vi "IO Docs.vi"(6 "OffsetGain":dbl[](array[numeric]), 7 "User Creds":T1, 8 "Error In":errorcluster, 9 "Digital IO":bool[](array[boolean]), 11 "Analog IO":dbl[](array[numeric])) -> (0 "Error Out":errorcluster, 1 "GXVALS Output":T3, 3 "Analog IO Out":dbl[](array[numeric]), 4 "BIAS DIFF Out":T2 {"DIFF" step=10.0; "BIAS" step=10.0}, 5 "OffsetGain Out":dbl[](array[numeric]))   [LabVIEW 2023]
uses:
  AnalogIOAll.ctl
  AnalogIOsingle.ctl
  biasdiff.ctl
  gridvals.ctl
  UserCredentials.ctl
  QSM - IODocs/Controls/State Machine Message.ctl
  QSM - IODocs/Controls/Message Queue Element Position.ctl
  QSM - IODocs/QSM - IODocs.lvlib
panel:
  in  "CLOSE":bool
  in  "GXVALS":T3
  in  "BIAS DIFF":T2 {"DIFF" step=10.0; "BIAS" step=10.0}
  out "DIO Cluster":T4
  in  "Analog IO Cluster":T5
  # "ANALOG I/O"
  # "GRID TANK VALUES"
  # "DIGITAL I/O"
  # "OFFSET"
  # "GAIN"
  # "OFFSET"
  # "GAIN"
  # "GAIN"
  # "OFFSET"
  # "GAIN"
  # "OFFSET"
  # "GAIN"
  # "OFFSET"
  # "GAIN"
  # "GAIN"
  # "OFFSET"
  # "GAIN"
  # "remKVSP"
  # "remKVrdg"
  # "remMASP"
  # "remMArdg"
  # "remEfDrSP"
  # "remEfDrRdg"
  # "remIfrdg"
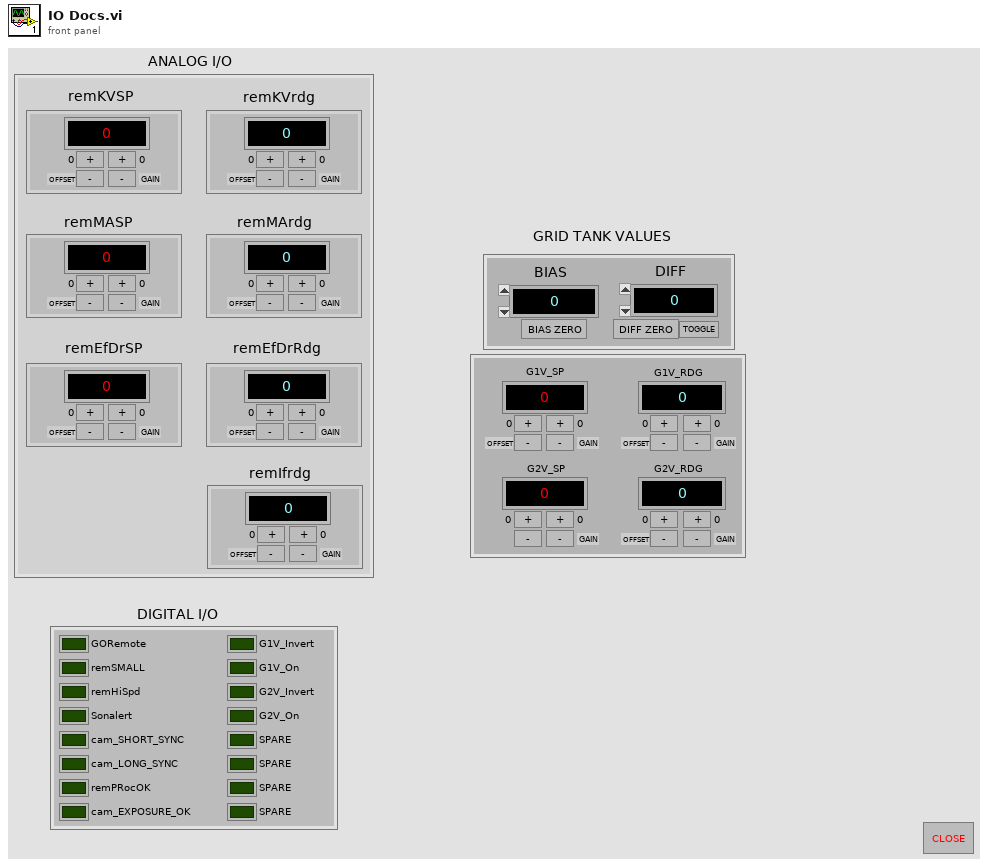
[diagram p1: front panel]
types:
  T1 = typedef "UserCredentials.ctl" = cluster{"Badge Number":string, "Name":string, "Access":enum16{"", "Operator", "Admin", "Engineer"}}
  T2 = typedef "biasdiff.ctl" = cluster{"BIAS":dbl, "BIAS_ZER":bool, "BIAS_ZER 2":bool, "DIFF_TOGGLE":bool, "DIFF":dbl}
  T3 = typedef "gridvals.ctl" = cluster{"G1V_SP":dbl, "G2V_SP":dbl, "G1V_RDG":dbl, "G2V_RDG":dbl, "G1sp offset up":bool, "G1sp offset down":bool, "G1sp gain up":bool, "G1sp gain down":bool, "G1rdg offset up":bool, "G1rdg offset down":bool, "G1rdg gain up":bool, "G1rdg gain down":bool, "G2sp offset up":bool, "G2sp offset down":bool, "G2sp gain up":bool, "G2sp gain down":bool, "G2rdg offset up":bool, "G2rdg offset down":bool, "G2rdg gain up":bool, "G2rdg gain down":bool, "g1spoffset":dbl, "g1spgain":dbl, "g2spoffset":dbl, "g2spgain":dbl, "g1rdgoffset":dbl, "g1rdggain":dbl, "g2rdgoffset":dbl, "g2rdggain":dbl}
  T4 = cluster{"GORemote":bool, "remSMALL":bool, "remHiSpd":bool, "Sonalert":bool, "cam_SHORT_SYNC":bool, "cam_LONG_SYNC":bool, "remPRocOK":bool, "cam_EXPOSURE_OK":bool, "G1V_Invert":bool, "G1V_On":bool, "G2V_Invert":bool, "G2V_On":bool, "SPARE":bool, "SPARE":bool, "SPARE":bool, "SPARE":bool}
  T5 = typedef "AnalogIOAll.ctl" = cluster{"AIO Cluster remKVSP":T6, "AIO Cluster remKVrdg":T6, "AIO Cluster remMASP":T6, "AIO Cluster remMArdg":T6, "AIO Cluster remEfDrSP":T6, "AIO Cluster remEfDrRdg":T6, "AIO Cluster remIfrdg":T6}
  T6 = typedef "AnalogIOsingle.ctl" = cluster{"I/O":dbl, "IO offset up":bool, "IO offset down":bool, "IO gain up":bool, "IO gain down":bool, "IOspoffset":dbl, "IOspgain":dbl}
  T7 = typedef "QSM - IODocs.lvlib/State Machine Message.ctl" = enum16{"Initialize", "Handle Error", "Exit"}
  T8 = cluster{"Value[0]":dbl, "Value[1]":dbl, "Value[2]":dbl, "Value[3]":dbl, "Value[4]":dbl, "Value[5]":dbl, "Value[6]":dbl, "Value[7]":dbl, "Value[8]":dbl, "Value[9]":dbl, "Value[10]":dbl, "Value[11]":dbl, "Value[12]":dbl, "Value[13]":dbl, "Value[14]":dbl, "Value[15]":dbl, "Value[16]":dbl, "Value[17]":dbl, "Value[18]":dbl, "Value[19]":dbl, "Value[20]":dbl, "Value[21]":dbl}
  T9 = cluster{"Value[0]":bool, "Value[1]":bool, "Value[2]":bool, "Value[3]":bool, "Value[4]":bool, "Value[5]":bool, "Value[6]":bool, "Value[7]":bool, "Value[8]":bool, "Value[9]":bool, "Value[10]":bool, "Value[11]":bool, "Value[12]":bool, "Value[13]":bool, "Value[14]":bool, "Value[15]":bool}
  T10 = enum8{"Enabled", "Disabled", "Disabled and Grayed Out"}
  T11 = cluster{"G1V_SP":dbl, "G2V_SP":dbl, "G1V_RDG":dbl, "G2V_RDG":dbl, "G1sp offset up":bool, "G1sp offset down":bool, "G1sp gain up":bool, "G1sp gain down":bool, "G1rdg offset up":bool, "G1rdg offset down":bool, "G1rdg gain up":bool, "G1rdg gain down":bool, "G2sp offset up":bool, "G2sp offset down":bool, "G2sp gain up":bool, "G2sp gain down":bool, "G2rdg offset up":bool, "G2rdg offset down":bool, "G2rdg gain up":bool, "G2rdg gain down":bool, "g1spoffset":dbl, "g1spgain":dbl, "g2spoffset":dbl, "g2spgain":dbl, "g1rdgoffset":dbl, "g1rdggain":dbl, "g2rdgoffset":dbl, "g2rdggain":dbl}
  T12 = cluster{"Value[0]":dbl, "Value[1]":dbl, "Value[2]":dbl, "Value[3]":dbl, "Value[4]":dbl, "Value[5]":dbl, "Value[6]":dbl, "Value[7]":dbl, "Value[8]":dbl, "Value[9]":dbl, "Value[10]":dbl}
  T13 = typedef "QSM - IODocs.lvlib/Message Queue Element Position.ctl" = enum16{"Front", "Back"}
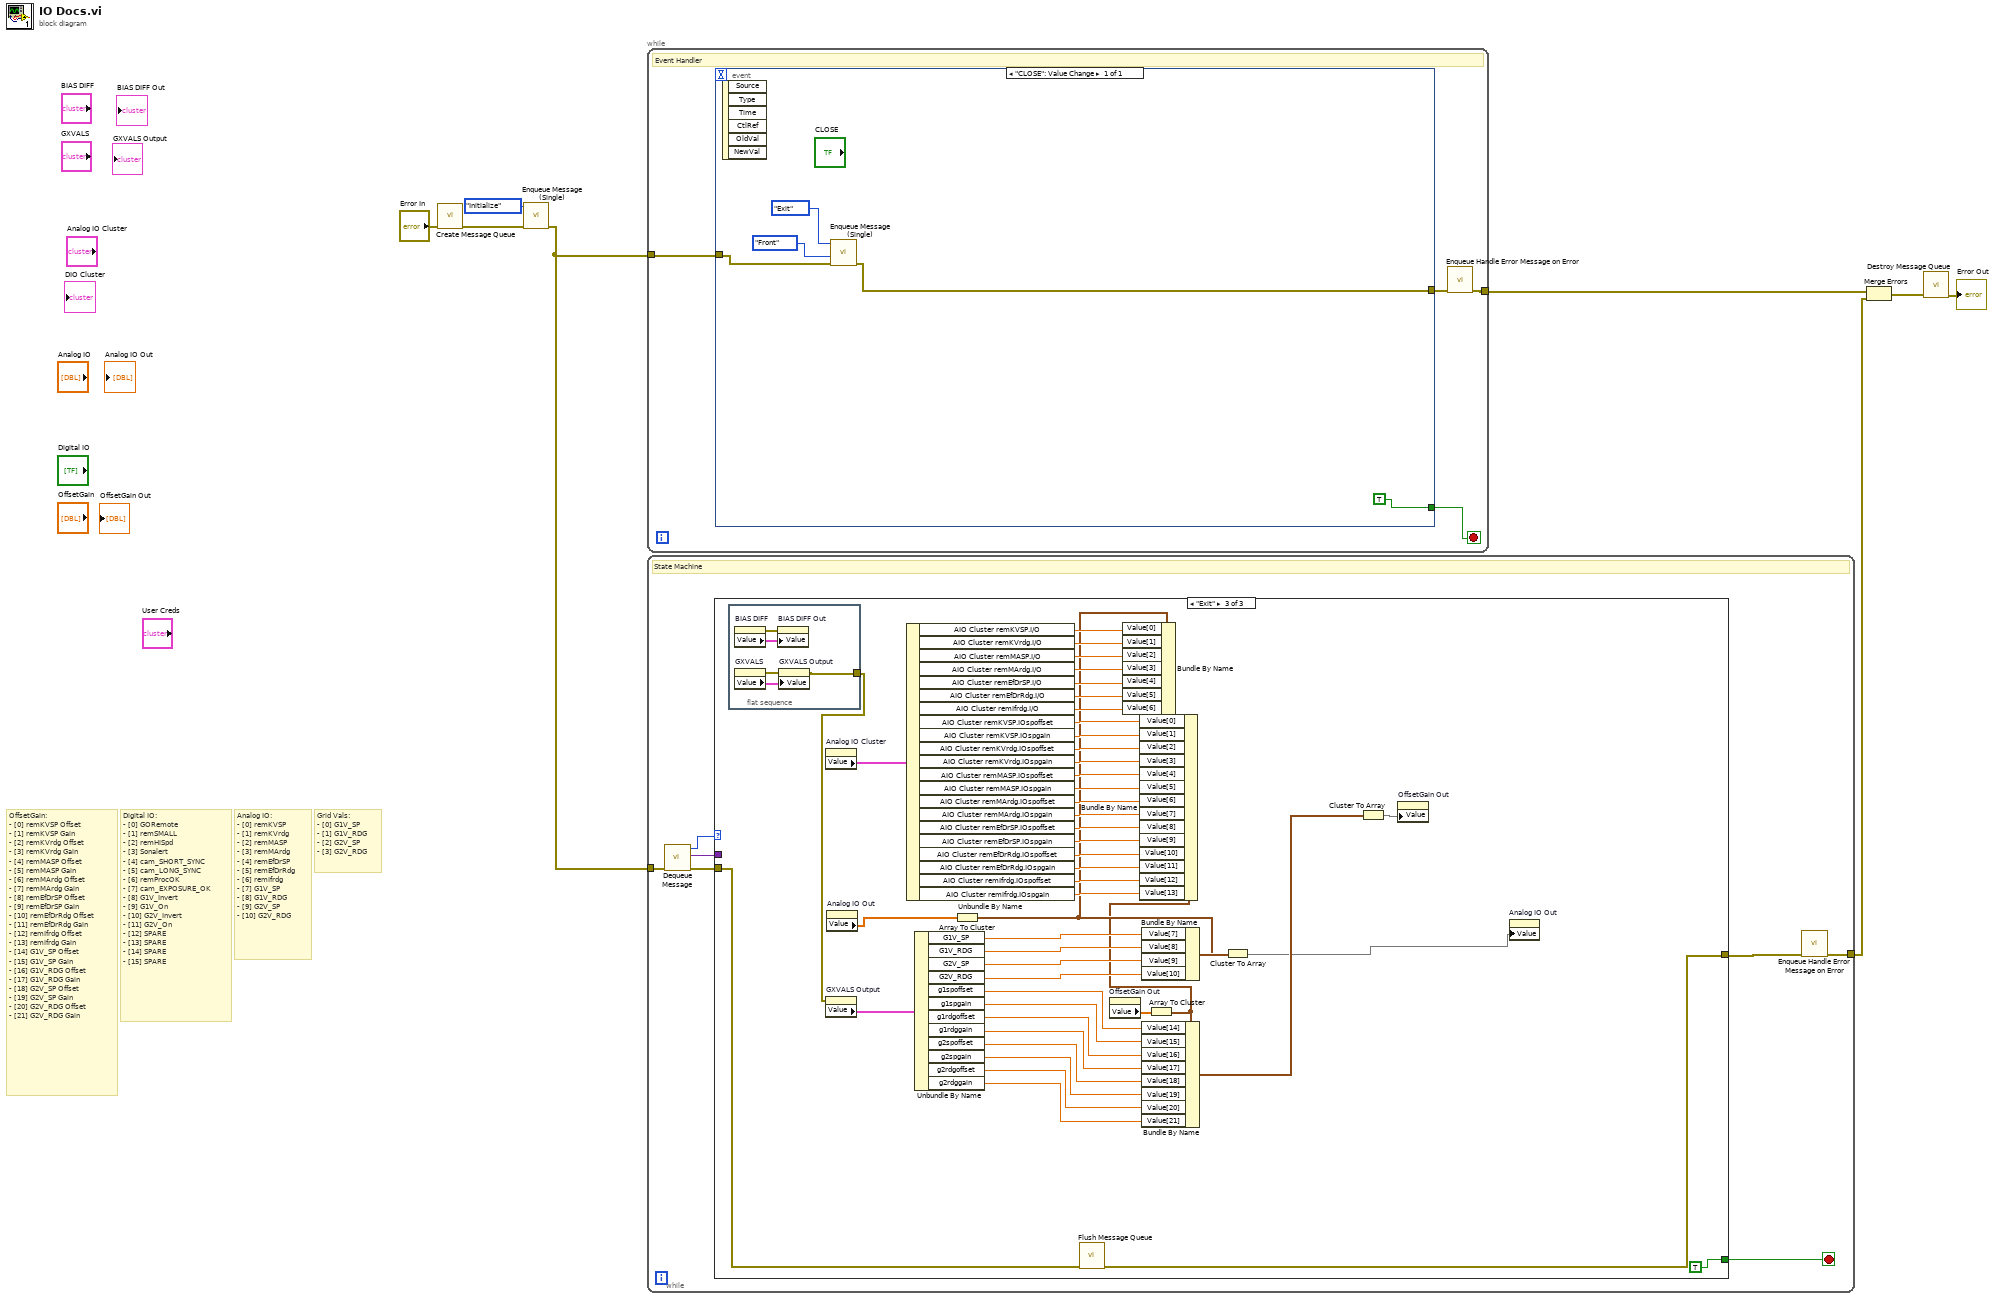
[diagram p0: block diagram]
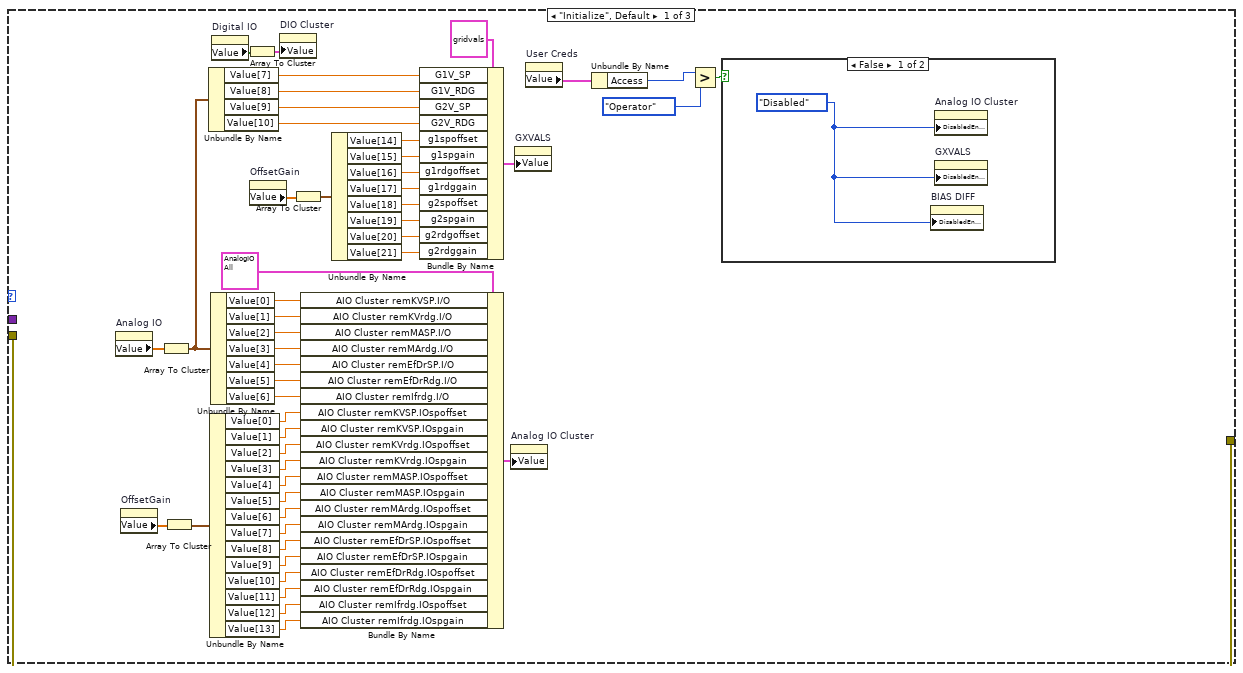
[diagram p2: hidden frame]
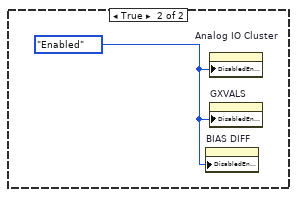
[diagram p3: hidden frame]
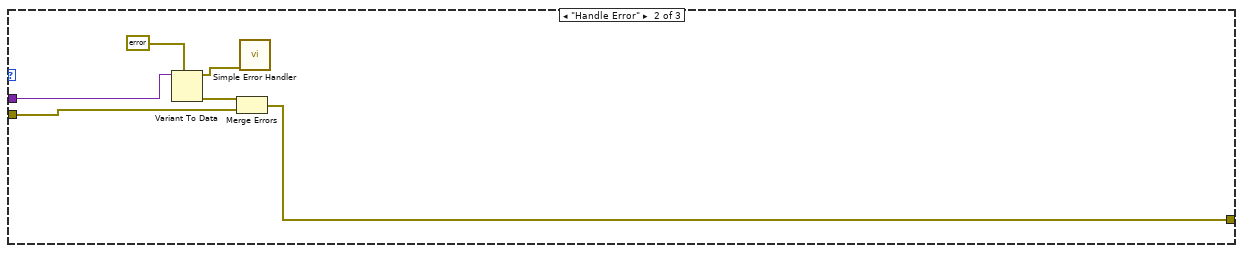
[diagram p4: hidden frame]
diagram:
  # "OffsetGain:\n- [0] remKVSP Offset\n- [1] remKVSP Gain\n- [2] remKVrdg Offset\n- [3] remKVrdg Gain\n- [4] remMASP Offset\n- [5] remMASP Gain\n- [6] remMArdg Offset\n- [7] remMArdg Gain\n- [8] remEfDrSP Offset\n- [9] remEfDrSP Gain\n- [10] remEfDrRdg Offset\n- [11] remEfDrRdg Gain\n- [12] remIfrdg Offset\n- [13] remIfrdg Gain\n- [14] G1V_SP Offset\n- [15] G1V_SP Gain\n- [16] G1V_RDG Offset\n- [17] G1V_RDG Gain\n- [18] G2V_SP Offset\n- [19] G2V_SP Gain\n- [20] G2V_RDG Offset\n- [21] G2V_RDG Gain"
  # "Digital IO:\n- [0] GORemote\n- [1] remSMALL\n- [2] remHiSpd\n- [3] Sonalert\n- [4] cam_SHORT_SYNC\n- [5] cam_LONG_SYNC\n- [6] remProcOK\n- [7] cam_EXPOSURE_OK\n- [8] G1V_Invert\n- [9] G1V_On\n- [10] G2V_Invert\n- [11] G2V_On\n- [12] SPARE\n- [13] SPARE\n- [14] SPARE\n- [15] SPARE"
  # "Grid Vals:\n- [0] G1V_SP\n- [1] G1V_RDG\n- [2] G2V_SP\n- [3] G2V_RDG"
  # "Analog IO:\n- [0] remKVSP\n- [1] remKVrdg\n- [2] remMASP\n- [3] remMArdg\n- [4] remEfDrSP\n- [5] remEfDrRdg\n- [6] remIfrdg\n- [7] G1V_SP\n- [8] G1V_RDG\n- [9] G2V_SP\n- [10] G2V_RDG"
  n1 = call "Create Message Queue.vi"("Error In"="Error In") -> ("Error Out"=w7:errorcluster)  [unwired: 10 in]
  n2 = call "Enqueue Message (Single).vi"("Error In"=w7, "State Machine Message"=State_Machine_Message."Initialize") -> ("Error Out"=w1:errorcluster)  [unwired: 9 in]
  n3 = while {
    tunnel: [w14] -> w5
    tunnel: w1 -> [w9]
    stop <- w15 stop-if-true
    # "State Machine"
    n4 = call "Dequeue Message.vi"("Error In"=w9) -> ("Error Out"=w13:errorcluster, "Data"=w11:variant, "State Machine Message"=w12:T7)  [unwired: 8 in]
    n5 = case shown="\"Exit\"" w12 {
      tunnel: [_ _ TRUE] -> w15
      tunnel: w13 -> [w65 w70 w120]
      tunnel: w11 -> [_ w69 _]
      tunnel: [w65 w68 w119] -> w10
      frame "Initialize", Default {
        n6 = property on="Analog IO" class="Arr (strict)"() -> ("Value"=w64:dbl[])  [unwired: 2 in, 2 out]
        n7 = property on="OffsetGain" class="Arr (strict)"() -> ("Value"=w38:dbl[])  [unwired: 2 in, 2 out]
        n8 = Array To Cluster(array=w64) -> (cluster=w22:T8)
        n9 = Array To Cluster(array=w38) -> (cluster=w37:T8)
        n10 = Unbundle By Name(w22) -> ("Value[7]"=w58:dbl, "Value[8]"=w57:dbl, "Value[9]"=w21:dbl, "Value[10]"=w20:dbl)
        n11 = Unbundle By Name(w37) -> ("Value[0]"=w36:dbl, "Value[1]"=w35:dbl, "Value[2]"=w34:dbl, "Value[3]"=w33:dbl, "Value[4]"=w32:dbl, "Value[5]"=w31:dbl, "Value[6]"=w30:dbl, "Value[7]"=w29:dbl, "Value[8]"=w28:dbl, "Value[9]"=w27:dbl, "Value[10]"=w26:dbl, "Value[11]"=w25:dbl, "Value[12]"=w24:dbl, "Value[13]"=w23:dbl)
        n12 = Unbundle By Name(w22) -> ("Value[0]"=w45:dbl, "Value[1]"=w44:dbl, "Value[2]"=w43:dbl, "Value[3]"=w42:dbl, "Value[4]"=w41:dbl, "Value[5]"=w40:dbl, "Value[6]"=w39:dbl)
        n13 = property on="Digital IO" class="Arr (strict)"() -> ("Value"=w61:bool[])  [unwired: 2 in, 2 out]
        n14 = Array To Cluster(array=w61) -> (cluster=w60:T9)
        n15 = property on="OffsetGain" class="Arr (strict)"() -> ("Value"=w56:dbl[])  [unwired: 2 in, 2 out]
        n16 = property on="DIO Cluster" class="Clust (strict)"("Value"=w60) -> ()  [unwired: 2 in, 2 out]
        n17 = Array To Cluster(array=w56) -> (cluster=w55:T8)
        n18 = Bundle By Name(cluster=T5 {"AIO Cluster remKVSP"={"I/O"=0.0, "IO offset up"=FALSE, "IO offset down"=FALSE, "IO gain up"=FALSE, "IO gain down"=FALSE, "IOspoffset"=0.0, "IOspgain"=0.0}, "AIO Cluster remKVrdg"={"I/O"=0.0, "IO offset up"=FALSE, "IO offset down"=FALSE, "IO gain up"=FALSE, "IO gain down"=FALSE, "IOspoffset"=0.0, "IOspgain"=0.0}, "AIO Cluster remMASP"={"I/O"=0.0, "IO offset up"=FALSE, "IO offset down"=FALSE, "IO gain up"=FALSE, "IO gain down"=FALSE, "IOspoffset"=0.0, "IOspgain"=0.0}, "AIO Cluster remMArdg"={"I/O"=0.0, "IO offset up"=FALSE, "IO offset down"=FALSE, "IO gain up"=FALSE, "IO gain down"=FALSE, "IOspoffset"=0.0, "IOspgain"=0.0}, "AIO Cluster remEfDrSP"={"I/O"=0.0, "IO offset up"=FALSE, "IO offset down"=FALSE, "IO gain up"=FALSE, "IO gain down"=FALSE, "IOspoffset"=0.0, "IOspgain"=0.0}, "AIO Cluster remEfDrRdg"={"I/O"=0.0, "IO offset up"=FALSE, "IO offset down"=FALSE, "IO gain up"=FALSE, "IO gain down"=FALSE, "IOspoffset"=0.0, "IOspgain"=0.0}, "AIO Cluster remIfrdg"={"I/O"=0.0, "IO offset up"=FALSE, "IO offset down"=FALSE, "IO gain up"=FALSE, "IO gain down"=FALSE, "IOspoffset"=0.0, "IOspgain"=0.0}} ("Analog IO Cluster"), "AIO Cluster remKVSP.I/O"=w45, "AIO Cluster remKVrdg.I/O"=w44, "AIO Cluster remMASP.I/O"=w43, "AIO Cluster remMArdg.I/O"=w42, "AIO Cluster remEfDrSP.I/O"=w41, "AIO Cluster remEfDrRdg.I/O"=w40, "AIO Cluster remIfrdg.I/O"=w39, "AIO Cluster remKVSP.IOspoffset"=w36, "AIO Cluster remKVSP.IOspgain"=w35, "AIO Cluster remKVrdg.IOspoffset"=w34, "AIO Cluster remKVrdg.IOspgain"=w33, "AIO Cluster remMASP.IOspoffset"=w32, "AIO Cluster remMASP.IOspgain"=w31, "AIO Cluster remMArdg.IOspoffset"=w30, "AIO Cluster remMArdg.IOspgain"=w29, "AIO Cluster remEfDrSP.IOspoffset"=w28, "AIO Cluster remEfDrSP.IOspgain"=w27, "AIO Cluster remEfDrRdg.IOspoffset"=w26, "AIO Cluster remEfDrRdg.IOspgain"=w25, "AIO Cluster remIfrdg.IOspoffset"=w24, "AIO Cluster remIfrdg.IOspgain"=w23) -> (w63:T5)
        n19 = Unbundle By Name(w55) -> ("Value[14]"=w54:dbl, "Value[15]"=w53:dbl, "Value[16]"=w52:dbl, "Value[17]"=w51:dbl, "Value[18]"=w50:dbl, "Value[19]"=w49:dbl, "Value[20]"=w48:dbl, "Value[21]"=w47:dbl)
        n20 = Bundle By Name(cluster=T3 {"G1V_SP"=0.0, "G2V_SP"=0.0, "G1V_RDG"=0.0, "G2V_RDG"=0.0, "G1sp offset up"=FALSE, "G1sp offset down"=FALSE, "G1sp gain up"=FALSE, "G1sp gain down"=FALSE, "G1rdg offset up"=FALSE, "G1rdg offset down"=FALSE, "G1rdg gain up"=FALSE, "G1rdg gain down"=FALSE, "G2sp offset up"=FALSE, "G2sp offset down"=FALSE, "G2sp gain up"=FALSE, "G2sp gain down"=FALSE, "G2rdg offset up"=FALSE, "G2rdg offset down"=FALSE, "G2rdg gain up"=FALSE, "G2rdg gain down"=FALSE, "g1spoffset"=0.0, "g1spgain"=0.0, "g2spoffset"=0.0, "g2spgain"=0.0, "g1rdgoffset"=0.0, "g1rdggain"=0.0, "g2rdgoffset"=0.0, "g2rdggain"=0.0} ("GXVALS"), "G1V_SP"=w58, "G1V_RDG"=w57, "G2V_SP"=w21, "G2V_RDG"=w20, "g1spoffset"=w54, "g1spgain"=w53, "g1rdgoffset"=w52, "g1rdggain"=w51, "g2spoffset"=w50, "g2spgain"=w49, "g2rdgoffset"=w48, "g2rdggain"=w47) -> (w46:T3)
        n21 = property on="Analog IO Cluster" class="Clust (strict)"("Value"=w63) -> ()  [unwired: 2 in, 2 out]
        n22 = property on="GXVALS" class="Clust (strict)"("Value"=w46) -> ()  [unwired: 2 in, 2 out]
        n23 = property on="User Creds" class="Clust (strict)"() -> ("Value"=w18:T1)  [unwired: 2 in, 2 out]
        n24 = Unbundle By Name(w18) -> ("Access"=w17:enum16{"", "Operator", "Admin", "Engineer"})
        n25 = Greater?(x=w17, y=enum16{"", "Operator", "Admin", "Engineer"}."Operator") -> (0:w19:bool)
        n26 = case shown="False" w19 {
          frame False {
            w66 = T10."Disabled" ("Disabled")
            n27 = property on="BIAS DIFF" class="Clust (strict)"("DisabledEnum"=w66) -> ()  [unwired: 2 in, 2 out]
            n28 = property on="Analog IO Cluster" class="Clust (strict)"("DisabledEnum"=w66) -> ()  [unwired: 2 in, 2 out]
            n29 = property on="GXVALS" class="Clust (strict)"("DisabledEnum"=w66) -> ()  [unwired: 2 in, 2 out]
          }
          frame True {
            w67 = T10."Enabled" ("Disabled")
            n30 = property on="BIAS DIFF" class="Clust (strict)"("DisabledEnum"=w67) -> ()  [unwired: 2 in, 2 out]
            n31 = property on="Analog IO Cluster" class="Clust (strict)"("DisabledEnum"=w67) -> ()  [unwired: 2 in, 2 out]
            n32 = property on="GXVALS" class="Clust (strict)"("DisabledEnum"=w67) -> ()  [unwired: 2 in, 2 out]
          }
        }
      }
      frame "Handle Error" {
        n33 = Variant To Data(type=errorcluster {"status"=FALSE, "code"=0, "source"=""} ("Error In"), Variant=w69) -> (data=w71:errorcluster, error out=w72:errorcluster)  [unwired: 1 in]
        n34 = Merge Errors(w72, w70) -> (w68:errorcluster)
        n35 = call <vilib>:"Simple Error Handler.vi"("error in (no error)"=w71) -> ()  [unwired: 4 in, 5 out]
      }
      frame "Exit" {
        n36 = flat-sequence {
          tunnel: [w121] -> w76
          frame #0 {
            n37 = property on="BIAS DIFF" class="Clust (strict)"() -> (error out=w125:errorcluster, "Value"=w124:T2)  [unwired: 2 in, 1 out]
            n38 = property on="GXVALS" class="Clust (strict)"() -> (error out=w123:errorcluster, "Value"=w122:T3)  [unwired: 2 in, 1 out]
            n39 = property on="BIAS DIFF Out" class="Clust (strict)"(error in=w125, "Value"=w124) -> ()  [unwired: 1 in, 2 out]
            n40 = property on="GXVALS Output" class="Clust (strict)"(error in=w123, "Value"=w122) -> (error out=w121:errorcluster)  [unwired: 1 in, 1 out]
          }
        }
        n41 = property on="Analog IO Cluster" class="Clust (strict)"() -> ("Value"=w117:T5)  [unwired: 2 in, 2 out]
        n42 = property on="GXVALS Output" class="Clust (strict)"(error in=w76) -> ("Value"=w116:T11)  [unwired: 1 in, 2 out]
        n43 = property on="Analog IO Out" class="Arr (strict)"() -> ("Value"=w79:dbl[])  [unwired: 2 in, 2 out]
        n44 = Unbundle By Name(w117) -> ("AIO Cluster remKVSP.I/O"=w101:dbl, "AIO Cluster remKVrdg.I/O"=w100:dbl, "AIO Cluster remMASP.I/O"=w99:dbl, "AIO Cluster remMArdg.I/O"=w98:dbl, "AIO Cluster remEfDrSP.I/O"=w97:dbl, "AIO Cluster remEfDrRdg.I/O"=w96:dbl, "AIO Cluster remIfrdg.I/O"=w95:dbl, "AIO Cluster remKVSP.IOspoffset"=w115:dbl, "AIO Cluster remKVSP.IOspgain"=w114:dbl, "AIO Cluster remKVrdg.IOspoffset"=w113:dbl, "AIO Cluster remKVrdg.IOspgain"=w112:dbl, "AIO Cluster remMASP.IOspoffset"=w111:dbl, "AIO Cluster remMASP.IOspgain"=w110:dbl, "AIO Cluster remMArdg.IOspoffset"=w109:dbl, "AIO Cluster remMArdg.IOspgain"=w108:dbl, "AIO Cluster remEfDrSP.IOspoffset"=w107:dbl, "AIO Cluster remEfDrSP.IOspgain"=w106:dbl, "AIO Cluster remEfDrRdg.IOspoffset"=w105:dbl, "AIO Cluster remEfDrRdg.IOspgain"=w104:dbl, "AIO Cluster remIfrdg.IOspoffset"=w103:dbl, "AIO Cluster remIfrdg.IOspgain"=w102:dbl)
        n45 = Unbundle By Name(w116) -> ("G1V_SP"=w94:dbl, "G1V_RDG"=w93:dbl, "G2V_SP"=w92:dbl, "G2V_RDG"=w91:dbl, "g1spoffset"=w90:dbl, "g1spgain"=w89:dbl, "g1rdgoffset"=w88:dbl, "g1rdggain"=w87:dbl, "g2spoffset"=w86:dbl, "g2spgain"=w85:dbl, "g2rdgoffset"=w84:dbl, "g2rdggain"=w83:dbl)
        n46 = Array To Cluster(array=w79) -> (cluster=w81:T12)
        n47 = call "Flush Message Queue.vi"("Error In"=w120) -> ("Error Out"=w119:errorcluster)  [unwired: 9 in, 1 out]
        n48 = property on="OffsetGain Out" class="Arr (strict)"() -> ("Value"=w78:dbl[])  [unwired: 2 in, 2 out]
        n49 = Bundle By Name(cluster=w81, "Value[0]"=w101, "Value[1]"=w100, "Value[2]"=w99, "Value[3]"=w98, "Value[4]"=w97, "Value[5]"=w96, "Value[6]"=w95) -> ()  [unwired: 1 out]
        n50 = Bundle By Name(cluster=w81, "Value[7]"=w94, "Value[8]"=w93, "Value[9]"=w92, "Value[10]"=w91) -> (w82:T12)
        n51 = Array To Cluster(array=w78) -> (cluster=w80:T8)
        n52 = Bundle By Name(cluster=w80, "Value[0]"=w115, "Value[1]"=w114, "Value[2]"=w113, "Value[3]"=w112, "Value[4]"=w111, "Value[5]"=w110, "Value[6]"=w109, "Value[7]"=w108, "Value[8]"=w107, "Value[9]"=w106, "Value[10]"=w105, "Value[11]"=w104, "Value[12]"=w103, "Value[13]"=w102) -> ()  [unwired: 1 out]
        n53 = Bundle By Name(cluster=w80, "Value[14]"=w90, "Value[15]"=w89, "Value[16]"=w88, "Value[17]"=w87, "Value[18]"=w86, "Value[19]"=w85, "Value[20]"=w84, "Value[21]"=w83) -> (w75:T8)
        n54 = Cluster To Array(cluster=w82) -> (array=w74:dbl[])
        n55 = Cluster To Array(cluster=w75) -> (array=w77:dbl[])
        n56 = property on="OffsetGain Out" class="Arr (strict)"("Value"=w77) -> ()  [unwired: 2 in, 2 out]
        n57 = property on="Analog IO Out" class="Arr (strict)"("Value"=w74) -> ()  [unwired: 2 in, 2 out]
      }
    }
    n58 = call "Enqueue Handle Error Message on Error.vi"("Error In"=w10) -> ("Error Out"=w14:errorcluster)  [unwired: 10 in]
  }
  n59 = while {
    tunnel: w1 -> [w128]
    tunnel: [w127] -> w2
    stop <- w129 stop-if-true
    # "Event Handler"
    n60 = event shown="[0] \"CLOSE\": Value Change" {
      selector: _ -> [_]
      dyn-events: _ -> [_]
      timeout: _ -> [_]
      tunnel: [TRUE] -> w129
      tunnel: w128 -> [w133]
      tunnel: [w131] -> w126
      event "CLOSE": Value Change {
        n61 = event-data() -> ()  [unwired: 1 in, 6 out]
        n62 = call "Enqueue Message (Single).vi"("Error In"=w133, "Message Position"=Message_Queue_Element_Position."Front", "State Machine Message"=State_Machine_Message."Exit") -> ("Error Out"=w131:errorcluster)  [unwired: 8 in]
      }
    }
    n63 = call "Enqueue Handle Error Message on Error.vi"("Error In"=w126) -> ("Error Out"=w127:errorcluster)  [unwired: 10 in]
  }
  n64 = Merge Errors(w2, w5) -> (w4:errorcluster)
  n65 = call "Destroy Message Queue.vi"("Error In"=w4) -> ("Error Out"=→"Error Out":errorcluster)  [unwired: 10 in]
